vi "Read Job Description.vi"(11 "Build Job in":refnum<class "Build Job.lvclass">) -> (2 "Job Description":string)   [LabVIEW 2014, in "Build Job.lvclass"]
uses:
  Build Job.lvclass
  Build Job.lvclass/Build Job.ctl
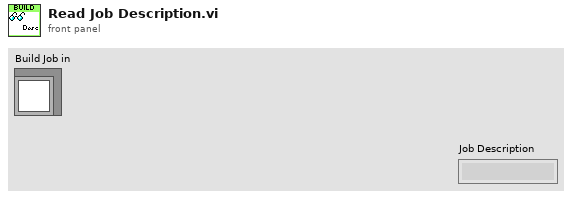
[diagram p1: front panel]
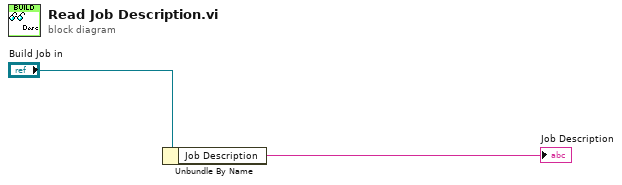
[diagram p0: block diagram]
diagram:
  n1 = Unbundle By Name("Build Job in") -> ("Job Description"=→"Job Description":string)
